vi "Deinitialize.vi"(8 "error in (no error)":errorcluster, 11 "Scanner reference":refnum<visa-resource-name>) -> (0 "error out":errorcluster)   [LabVIEW 2023, in "HoneywellScanner.lvlib"]
uses:
  HoneywellScanner.lvlib
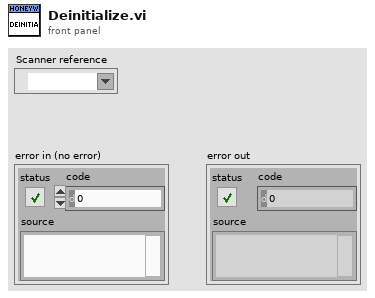
[diagram p1: front panel]
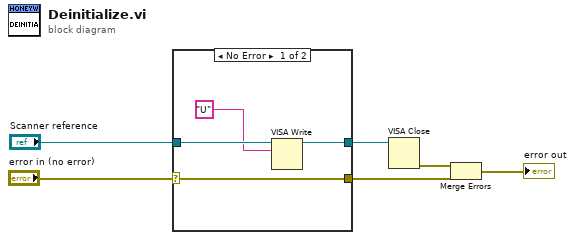
[diagram p0: block diagram]
diagram:
  n1 = case shown="No Error" "error in (no error)" {
    selector: "error in (no error)" -> [w7 w11]
    tunnel: [w10 w12] -> w6
    tunnel: "Scanner reference" -> [w9 w12]
    tunnel: [w7 w11] -> w3
    frame No Error {
      n2 = VISA Write(VISA resource name=w9, write buffer="U") -> (VISA resource name out=w10:refnum<visa-resource-name>)  [unwired: 1 in, 2 out]
    }
    frame Error {
    }
  }
  n3 = VISA Close(VISA resource name=w6) -> (error out=w2:errorcluster)  [unwired: 1 in]
  n4 = Merge Errors(w2, w3) -> (→"error out":errorcluster)
